vi "Basic.vi"() -> ()   [LabVIEW 2015]
panel:
  in  "C":dbl
  out "D":dbl
  in  "B":dbl
  in  "A":dbl
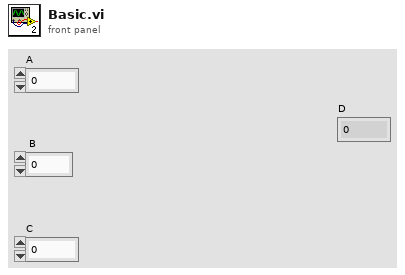
[diagram p1: front panel]
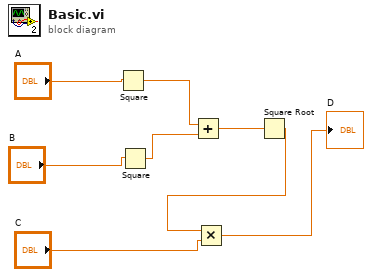
[diagram p0: block diagram]
diagram:
  n1 = Square(x="A") -> (x^2=w6:dbl)
  n2 = Square(x="B") -> (x^2=w4:dbl)
  n3 = Add(x=w6, y=w4) -> (x+y=w5:dbl)
  n4 = Square Root(x=w5) -> (sqrt(x)=w2:dbl)
  n5 = Multiply(x=w2, y="C") -> (x*y=→"D":dbl)
